vi "Set SMS Attributes.vi"(8 "error in (no error)":errorcluster, 10 "SMS Attributes":T1[](array[typedef]), 11 "SMS in":refnum<class "SMS.lvclass">) -> (0 "error out":errorcluster, 3 "SMS out":refnum<class "SMS.lvclass">)   [LabVIEW 2015, in "NI_AWS_SNS.lvlib" / "SMS.lvclass"]
doc: "The default settings for sending SMS messages from your account. You can set values for the following attribute names:\n\nMonthlySpendLimit – The maximum amount in USD that you are willing to spend each month to send SMS messages. When Amazon SNS determines that sending an SMS message would incur a cost that exceeds this limit, it stops sending SMS messages within minutes.\n\nImportant\nAmazon SNS stops sending SMS messages within minutes of the limit being crossed. During that interval, if you continue to send SMS messages, you will incur costs that exceed your limit.\nBy default, the spend limit is set to the maximum allowed by Amazon SNS. If you want to raise the limit, submit an SNS Limit Increase case. For New limit value, enter your desired monthly spend limit. In the Use Case Description field, explain that you are requesting an SMS monthly spend limit increase.\n\nDeliveryStatusIAMRole – The ARN of the IAM role that allows Amazon SNS to write logs about SMS deliveries in CloudWatch Logs. For each SMS message that you send, Amazon SNS writes a log that includes the message price, the success or failure status, the reason for failure (if the message failed), the message dwell time, and other information.\n\nDeliveryStatusSuccessSamplingRate – The percentage of successful SMS deliveries for which Amazon SNS will write logs in CloudWatch Logs. The value can be an integer from 0 - 100. For example, to write logs only for failed deliveries, set this value to 0. To write logs for 10% of your successful deliveries, set it to 10.\n\nDefaultSenderID – A string, such as your business brand, that is displayed as the sender on the receiving device. Support for sender IDs varies by country. The sender ID can be 1 - 11 alphanumeric characters, and it must contain at least one letter.\n\nDefaultSMSType – The type of SMS message that you will send by default. You can assign the following values:\n\nPromotional – (Default) Noncritical messages, such as marketing messages. Amazon SNS optimizes the message delivery to incur the lowest cost.\nTransactional – Critical messages that support customer transactions, such as one-time passcodes for multi-factor authentication. Amazon SNS optimizes the message delivery to achieve the highest reliability.\nUsageReportS3Bucket – The name of the Amazon S3 bucket to receive daily SMS usage reports from Amazon SNS. Each day, Amazon SNS will deliver a usage report as a CSV file to the bucket. The report includes the following information for each SMS message that was successfully delivered by your account:\n\nTime that the message was published (in UTC)\nMessage ID\nDestination phone number\nMessage type\nDelivery status\nMessage price (in USD)\nPart number (a message is split into multiple parts if it is too long for a single message)\nTotal number of parts"
uses:
  SMS.lvclass
  SMS Attribute Value Pair.ctl
  SMS Attribute.ctl
  Core/HTTP Request/Request Options.ctl
  Core/HTTP Request/Name Value Pair.ctl
  Core/HTTP Request/Region handling.ctl
  Core/HTTP Request/URL formatting.ctl
  Core/HTTP Request/HTTP Request.lvclass
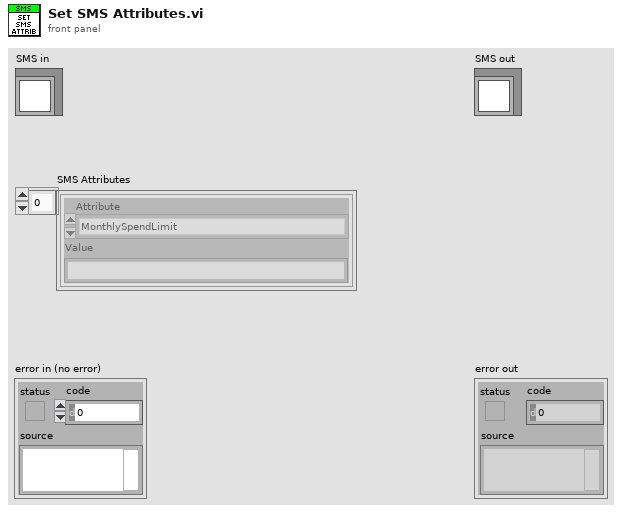
[diagram p1: front panel]
types:
  T1 = typedef "NI_AWS_SNS.lvlib/SMS.lvclass/SMS Attribute Value Pair.ctl" = cluster{"Attribute":T2, "Value":string}
  T2 = typedef "NI_AWS_SNS.lvlib/SMS.lvclass/SMS Attribute.ctl" = enum16{"MonthlySpendLimit", "DeliveryStatusIAMRole", "DeliveryStatusSuccessSamplingRate", "DefaultSenderID", "DefaultSMSType", "UsageReportS3Bucket"}
  T3 = typedef "NI_AWS_Core.lvlib/HTTP Request.lvclass/Name Value Pair.ctl" = cluster{"name":string, "value":string}
  T4 = typedef "NI_AWS_Core.lvlib/HTTP Request.lvclass/Request Options.ctl" = cluster{"request headers":T3[], "request parameters":T3[], "request body":string, "region handling":T5, "URL formatting":T6}
  T5 = typedef "NI_AWS_Core.lvlib/HTTP Request.lvclass/Region handling.ctl" = enum16{"use region everywhere", "use region (authentication only)", "use region (URL only)", "ignore region everwhere"}
  T6 = typedef "NI_AWS_Core.lvlib/HTTP Request.lvclass/URL formatting.ctl" = enum16{"region-", "region."}
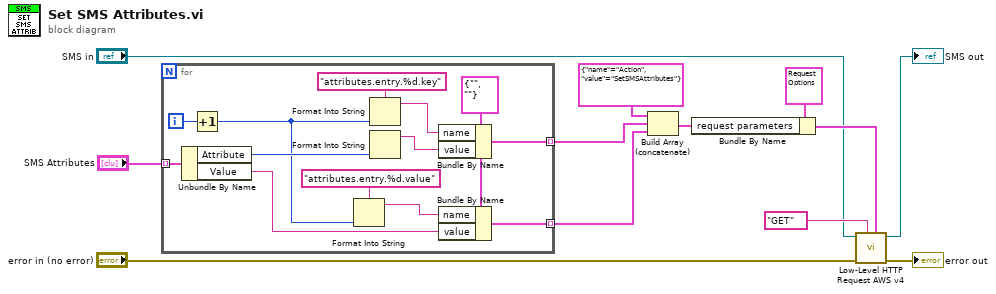
[diagram p0: block diagram]
diagram:
  n1 = for {
    tunnel: "SMS Attributes" -> [w21] mode=indexing
    tunnel: [w23] -> w6 mode=indexing
    tunnel: [w22] -> w5 mode=indexing
    i -> [w25]
    w24 = T3 {"name"="", "value"=""} ("element")
    n2 = Unbundle By Name(w21) -> ("Attribute"=w18:T2, "Value"=w16:string)
    n3 = Increment(x=w25) -> (x+1=w13:i32)
    n4 = Format Into String(format string="attributes.entry.%d.value", w13) -> (resulting string=w14:string)  [unwired: 2 in, 1 out]
    n5 = Format Into String(format string="attributes.entry.%d.key", w13) -> (resulting string=w19:string)  [unwired: 2 in, 1 out]
    n6 = Format Into String(w18) -> (resulting string=w17:string)  [unwired: 3 in, 1 out]
    n7 = Bundle By Name(cluster=w24, "name"=w19, "value"=w17) -> (w23:T3)
    n8 = Bundle By Name(cluster=w24, "name"=w14, "value"=w16) -> (w22:T3)
  }
  n9 = Build Array (concatenate)(T3 {"name"="Action", "value"="SetSMSAttributes"} ("Name Value Pair"), w6, w5) -> (w9:T3[])
  n10 = Bundle By Name(cluster=T4 {"request headers"=[], "request parameters"=[], "request body"="", "region handling"=enum."use region everywhere", "URL formatting"=enum."region."} ("Request Options"), "request parameters"=w9) -> (w4:T4)
  n11 = call "Low-Level HTTP Request AWS v4.vi"("Request Options"=w4, "HTTP-Verb"="GET", "error in (no error)"="error in (no error)", "AWS Core in"="SMS in") -> ("error out"=→"error out":errorcluster, "AWS Core out"=→"SMS out":refnum<class "SMS.lvclass">)  [unwired: 4 in, 2 out]
